vi "Teleop.vi"(10 "Match Info":T1={"Autonomous Elapsed Seconds"=0.0, "TeleOp Elapsed Seconds"=0.0, "Disabled Elapsed Seconds"=0.0, "Visited Autonomous"=FALSE, "Visited TeleOp"=FALSE, "Visited Disabled"=FALSE, "Autonomous Settings"={"Autonomous Style"=enum."Independent", "VI Refnum"=refnum}}, 11 "Call Context":T2) -> ()   [LabVIEW 2016]
doc: "This VI is called for each TeleOp packet received from the DS where the robot is not disabled. It is often used to read from the joysticks and update I/O or to update setpoints for timed control loops. It should complete and return within 20 milliseconds or it may miss DS packets."
uses:
  <vilib>/Rock Robotics/WPI/DriverStation/WPI_DriverStationDerivedRobotMode.ctl
  <vilib>/Rock Robotics/WPI/DriverStation/WPI_DriverStationMatch Info.ctl
  <vilib>/Rock Robotics/WPI/Solenoid/WPI_SolenoidValue.ctl
  <vilib>/Rock Robotics/WPI/Utilities/WPI_GetSetVariantRefNum.vi
  <vilib>/Rock Robotics/Network Tables/NT Read Boolean.vi
  <vilib>/Rock Robotics/Network Tables/NT Read Number.vi
  <vilib>/Rock Robotics/WPI/Solenoid/WPI_SolenoidSetEnum.vi
panel:
  in  "Reset Encoder":bool
  out "Moyenne encodeur":dbl
  out "Encodeur Droit":dbl
  out "Ecodeur Gauche":dbl
  out "Sample Slider 0":dbl(slide) scale=0.0..5.0
  out "Sample Boolean 1":bool
  out "Sample Boolean 0":bool
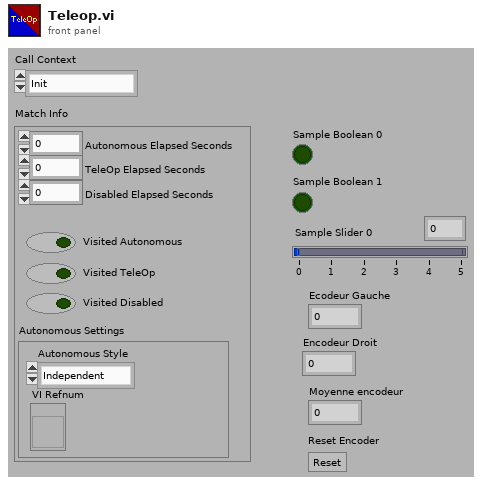
[diagram p1: front panel]
types:
  T1 = typedef "WPI_DriverStationMatch Info.ctl" = cluster{"Autonomous Elapsed Seconds":dbl, "TeleOp Elapsed Seconds":dbl, "Disabled Elapsed Seconds":dbl, "Visited Autonomous":bool, "Visited TeleOp":bool, "Visited Disabled":bool, "Autonomous Settings":cluster{"Autonomous Style":enum16{"Iterative", "Independent"}, "VI Refnum":refnum<vi>}}
  T2 = typedef "WPI_DriverStationDerivedRobotMode.ctl" = enum16{"Init", "Execute", "Stop"}
  T3 = typedef "WPI_SolenoidValue.ctl" = enum16{"Off", "On", "Forward", "Reverse"}
  T4 = typedef "WPI_JoystickDevRef.ctl" = cluster{"Device":T5}
  T5 = typedef "WPI_JoystickDeviceEnum.ctl" = enum16{"USB 0", "USB 1", "USB 2", "USB 3", "USB 4", "USB 5"}
  T6 = cluster{"Buttons[0]":bool, "Buttons[1]":bool, "Buttons[2]":bool, "Buttons[3]":bool, "Buttons[4]":bool, "Buttons[5]":bool, "Buttons[6]":bool, "Buttons[7]":bool, "Buttons[8]":bool}
  T7 = cluster{"Axes[0]":dbl, "Axes[1]":dbl, "Axes[2]":dbl, "Axes[3]":dbl, "Axes[4]":dbl, "Axes[5]":dbl, "Axes[6]":dbl, "Axes[7]":dbl, "Axes[8]":dbl}
  T8 = typedef "WPI_RobotDriveDevRef.ctl" = cluster{"DevStatus":errorcluster, "Motors[]":T9[], "Square Inputs":bool, "Max Output":dbl}
  T9 = typedef "WPI_MotorControlDeviceRef.ctl" = cluster{"DeviceStatus":errorcluster, "Type":T10, "PWM":cluster{"PWM Channel":T11, "DeadBand":T12}, "CAN":cluster{"Device Number":u8, "SetOutput VI Ref":variant, "GetOutput VI Ref":variant, "Enable VI Ref":variant, "Disable VI Ref":variant, "Data":variant}, "Invert":bool}
  T10 = typedef "WPI_MotorControlType.ctl" = enum16{"PWM", "CAN"}
  T11 = typedef "FPGA_DIOPWMChannel.ctl" = enum8{"PWM 0", "PWM 1", "PWM 2", "PWM 3", "PWM 4", "PWM 5", "PWM 6", "PWM 7", "PWM 8", "PWM 9", "PWM MXP 0", "PWM MXP 1", "PWM MXP 2", "PWM MXP 3", "PWM MXP 4", "PWM MXP 5", "PWM MXP 6", "PWM MXP 7", "PWM MXP 8", "PWM MXP 9", "Invalid"}
  T12 = typedef "WPI_PWMDeadband.ctl" = cluster{"Name":string, "maxPositivePwm":i32, "minPositivePwm":i32, "centerPwm":i32, "maxNegativePwm":i32, "minNegativePwm":i32, "angularRange":u16}
  T13 = typedef "WPI_SolenoidDevRef.ctl" = cluster{"DevStatus":errorcluster, "Pneumatics Control Module":u8, "Forward Solenoid Channel":T14, "Reverse Solenoid Channel":T14}
  T14 = typedef "WPI_SolenoidChannel.ctl" = enum8{"Solenoid 0", "Solenoid 1", "Solenoid 2", "Solenoid 3", "Solenoid 4", "Solenoid 5", "Solenoid 6", "Solenoid 7", "Invalid"}
  T15 = typedef "WPI_EncoderDevRef.ctl" = cluster{"DevStatus":errorcluster, "EncoderIndex":T16, "CounterIndex":T17, "DistancePerCount":dbl, "Decoding Type":T18}
  T16 = typedef "FPGA_EncoderIdx.ctl" = enum8{"Enc 0", "Enc 1", "Enc 2", "Enc 3", "Enc 4", "Enc 5", "Enc 6", "Enc 7", "Invalid"}
  T17 = typedef "FPGA_CounterCtrSystemIndex.ctl" = enum8{"Ctr 0", "Ctr 1", "Ctr 2", "Ctr 3", "Ctr 4", "Ctr 5", "Ctr 6", "Ctr 7", "Invalid"}
  T18 = typedef "WPI_EncoderType.ctl" = enum16{"1x", "2x", "4x"}
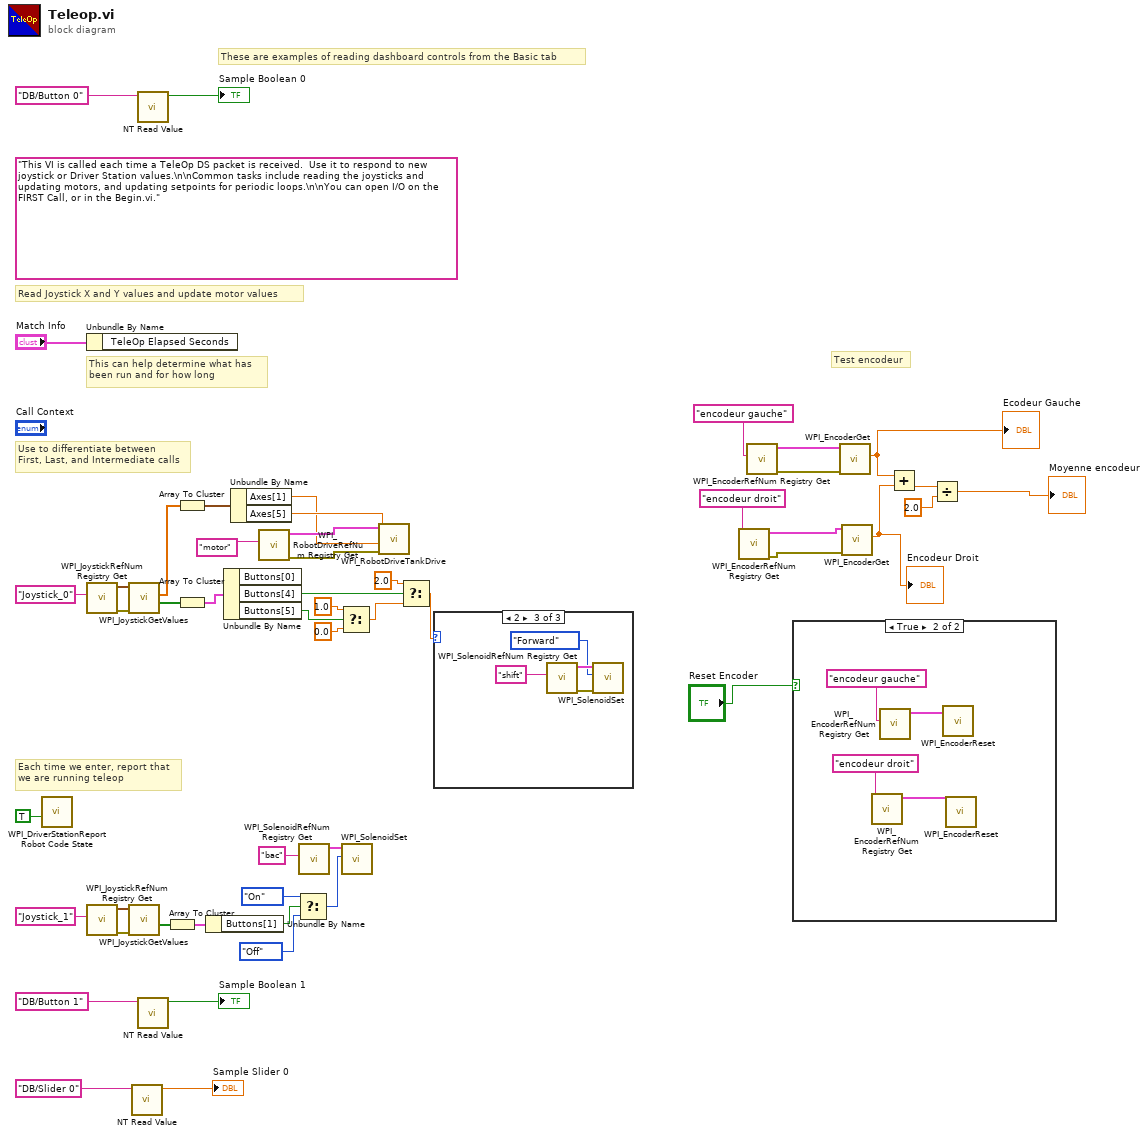
[diagram p0: block diagram]
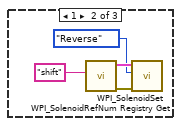
[diagram p4: hidden frame]
diagram:
  (unwired) "This VI is called each time a TeleOp DS packet is received.  Use it to respond to new joystick or Driver Station values.\n\nCommon tasks include reading the joysticks and updating motors, and updating setpoints for periodic loops.\n\nYou can open I/O on the FIRST Call, or in the Begin.vi."
  # "Test encodeur"
  # "These are examples of reading dashboard controls from the Basic tab"
  # "Each time we enter, report that\nwe are running teleop"
  # "Use to differentiate between\nFirst, Last, and Intermediate calls"
  # "This can help determine what has\nbeen run and for how long"
  # "Read Joystick X and Y values and update motor values"
  n1 = call <vilib>:"WPI_DriverStationReport Robot Code State.vi"("TeleOp"=TRUE ("Autonomous")) -> ()  [unwired: 10 in, 1 out]
  n2 = Unbundle By Name("Match Info") -> ()  [unwired: 1 out]
  n3 = call <vilib>:"WPI_JoystickRefNum Registry Get.vi"("refnum name"="Joystick_0") -> ("error out"=w30:errorcluster, "JoystickDevRef"=w48:T4)  [unwired: 1 in, 8 out]
  n4 = call <vilib>:"WPI_JoystickRefNum Registry Get.vi"("refnum name"="Joystick_1") -> ("error out"=w29:errorcluster, "JoystickDevRef"=w31:T4)  [unwired: 1 in, 8 out]
  n5 = call <vilib>:"WPI_JoystickGetValues.vi"("error in (no error)"=w30, "JoystickDevRef"=w48) -> ("Buttons"=w39:bool[], "Axes"=w40:dbl[])  [unwired: 5 in, 3 out]
  n6 = call <vilib>:"WPI_JoystickGetValues.vi"("error in (no error)"=w29, "JoystickDevRef"=w31) -> ("Buttons"=w28:bool[])  [unwired: 5 in, 4 out]
  n7 = call-poly <vilib>:"NT Read Value.vi"("Name"="DB/Slider 0" ("refnum name")) -> ("Numeric"=→"Sample Slider 0":dbl)  [unwired: 9 in, 1 out]
  n8 = call-poly <vilib>:"NT Read Value.vi"("Name"="DB/Button 0" ("refnum name")) -> ("Boolean"=→"Sample Boolean 0":bool)  [unwired: 9 in, 1 out]
  n9 = call-poly <vilib>:"NT Read Value.vi"("Name"="DB/Button 1" ("refnum name")) -> ("Boolean"=→"Sample Boolean 1":bool)  [unwired: 9 in, 1 out]
  n10 = Array To Cluster(array=w28) -> (cluster=w27:T6)
  n11 = Array To Cluster(array=w40) -> (cluster=w38:T7)
  n12 = Array To Cluster(array=w39) -> (cluster=w37:T6)
  n13 = Unbundle By Name(w27) -> ("Buttons[1]"=w26:bool)
  n14 = Unbundle By Name(w37) -> ("Buttons[4]"=w36:bool, "Buttons[5]"=w23:bool)  [unwired: 1 out]
  n15 = Unbundle By Name(w38) -> ("Axes[1]"=w13:dbl, "Axes[5]"=w14:dbl)
  n16 = call <vilib>:"WPI_RobotDriveRefNum Registry Get.vi"("refnum name"="motor") -> ("error out"=w33:errorcluster, "RobotDriveDevRef"=w34:T8)  [unwired: 9 in]
  n17 = Select(t=WPI_SolenoidValue."On" ("Value"), s=w26, f=WPI_SolenoidValue."Off" ("Value")) -> (s? t:f=w17:T3)
  n18 = call <vilib>:"WPI_SolenoidRefNum Registry Get.vi"("refnum name"="bac") -> ("SolenoidDevRef"=w18:T13)  [unwired: 9 in, 1 out]
  n19 = Select(t=1.0, s=w23, f=0.0) -> (s? t:f=w22:dbl)
  n20 = call-poly <vilib>:"WPI_SolenoidSet.vi"("Value"=w17, "SolenoidDevRef"=w18) -> ()  [unwired: 8 in, 2 out]
  n21 = call <vilib>:"WPI_RobotDriveTankDrive.vi"("error in (no error)"=w33, "Right axis value"=w13, "Left axis value"=w14, "RobotDriveDevRef"=w34) -> ()  [unwired: 5 in, 3 out]
  n22 = Select(t=2.0, s=w36, f=w22) -> (s? t:f=w25:dbl)
  n23 = case shown="2" w25 {
    frame 0, Default {
    }
    frame 1 {
      n24 = call <vilib>:"WPI_SolenoidRefNum Registry Get.vi"("refnum name"="shift") -> ("error out"=w53:errorcluster, "SolenoidDevRef"=w52:T13)  [unwired: 9 in]
      n25 = call-poly <vilib>:"WPI_SolenoidSet.vi"("error in (no error)"=w53, "Value"=WPI_SolenoidValue."Reverse", "SolenoidDevRef"=w52) -> ()  [unwired: 7 in, 2 out]
    }
    frame 2 {
      n26 = call <vilib>:"WPI_SolenoidRefNum Registry Get.vi"("refnum name"="shift") -> ("error out"=w57:errorcluster, "SolenoidDevRef"=w56:T13)  [unwired: 9 in]
      n27 = call-poly <vilib>:"WPI_SolenoidSet.vi"("error in (no error)"=w57, "Value"=WPI_SolenoidValue."Forward", "SolenoidDevRef"=w56) -> ()  [unwired: 7 in, 2 out]
    }
  }
  n28 = call <vilib>:"WPI_EncoderRefNum Registry Get.vi"("refnum name"="encodeur droit") -> ("error out"=w5:errorcluster, "EncoderDevRef"=w6:T15)  [unwired: 9 in]
  n29 = call <vilib>:"WPI_EncoderRefNum Registry Get.vi"("refnum name"="encodeur gauche") -> ("error out"=w7:errorcluster, "EncoderDevRef"=w8:T15)  [unwired: 9 in]
  n30 = case shown="True" "Reset Encoder" {
    frame False {
    }
    frame True {
      n31 = call <vilib>:"WPI_EncoderRefNum Registry Get.vi"("refnum name"="encodeur droit") -> ("EncoderDevRef"=w59:T15)  [unwired: 9 in, 1 out]
      n32 = call <vilib>:"WPI_EncoderRefNum Registry Get.vi"("refnum name"="encodeur gauche") -> ("EncoderDevRef"=w60:T15)  [unwired: 9 in, 1 out]
      n33 = call <vilib>:"WPI_EncoderReset.vi"("EncoderDevRef"=w60) -> ()  [unwired: 9 in, 2 out]
      n34 = call <vilib>:"WPI_EncoderReset.vi"("EncoderDevRef"=w59) -> ()  [unwired: 9 in, 2 out]
    }
  }
  n35 = call <vilib>:"WPI_EncoderGet.vi"("error in (no error)"=w7, "EncoderDevRef"=w8) -> ("Distance"=w4:dbl)  [unwired: 4 in, 5 out]
  "Ecodeur Gauche" <- w4
  n36 = call <vilib>:"WPI_EncoderGet.vi"("error in (no error)"=w5, "EncoderDevRef"=w6) -> ("Distance"=w3:dbl)  [unwired: 4 in, 5 out]
  "Encodeur Droit" <- w3
  n37 = Add(x=w4, y=w3) -> (x+y=w10:dbl)
  n38 = Divide(x=w10, y=2.0) -> (x/y=→"Moyenne encodeur":dbl)
